vi "Levenberg Marquardt Prep.vi"(0 "Structure":T1 {"?" format="%.2f"; "?" format="%.2f"; "Initial Guess Coefficient" format="%.2f"; "?" format="%.2f"; "X" format="%.2f"; "Parsed Formula copy"."Y Values" format="%.2f"; "Y Values" format="%.2f"; "Y" format="%.2f"; "Parsed Formula"."Y Values" format="%.2f"}, 1 "max iteration":i32=200) -> (2 "Covariance":dbl[][](array[numeric]) format="%.2f", 3 "Best Fit":dbl[](array[numeric]) format="%.2f", 4 "Best Fit Coefficients":dbl[](array[numeric]) format="%.2f", 5 "mse":dbl format="%.2e")   [LabVIEW 2017, in "NI_Gmath.lvlib"]
uses:
  NI_Gmath.lvlib
  Real Outer Product.vi
  Solve Linear Equations (single right hand).vi
  Solve Linear Equations By Cholesky.vi
  Real Matrix to Compact Array.vi
  Real Compact Tri-Matrix Linear Eqs.vi
  Solve Linear Eqs (General).vi
  Solve Linear Eqs (Gen, single right hand).vi
  Add - RM,RM.vi
  Multiply - RM,RM.vi
  Multiply - R,RM.vi
  Create Special Real Matrix.vi
  NI_AALPro.lvlib
  NI_AALBase.lvlib
  NI_Matrix.lvlib
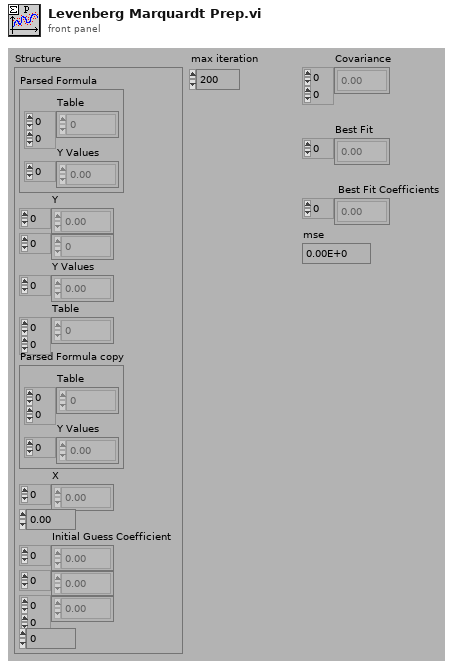
[diagram p1: front panel]
types:
  T1 = cluster{"Parsed Formula":cluster{"Table":i32[][], "Y Values":dbl[]}, "Y":dbl[], i32[], "Y Values":dbl[], "Table":i32[][], "Parsed Formula copy":cluster{"Table":i32[][], "Y Values":dbl[]}, "X":dbl[], dbl, "Initial Guess Coefficient":dbl[], dbl[], dbl[][], i32}
  T2 = enum32{"Identity", "Diagonal", "Toepliz", "Vandermonde", "Companion"}
  T3 = typedef "NI_Matrix.lvlib/RealMatrix.ctl" = dbl[][]
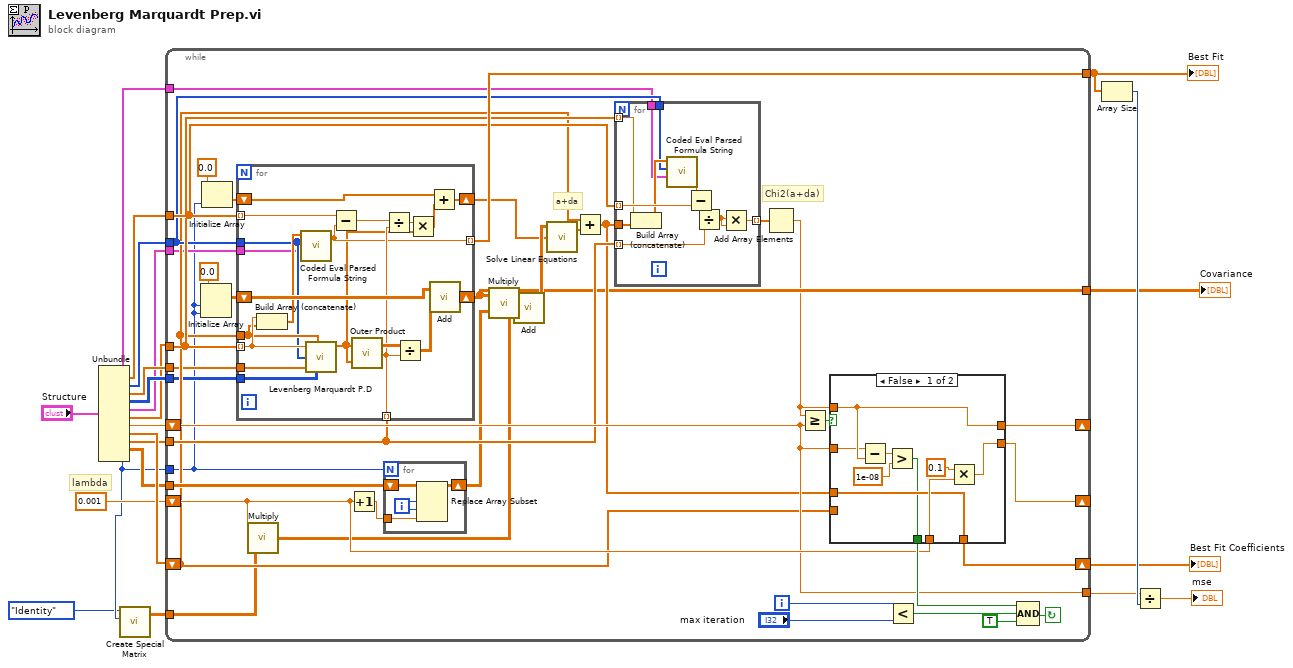
[diagram p0: block diagram]
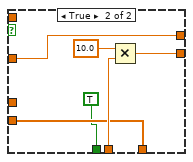
[diagram p2: hidden frame]
diagram:
  # "lambda"
  n1 = Unbundle("Structure") -> ("Parsed Formula"=w11:cluster{"Table":i32[][], "Y Values":dbl[]}, "Y"=w12:dbl[], w13:i32[], "Y Values"=w20:dbl[], "Table"=w19:i32[][], "Parsed Formula copy"=w14:cluster{"Table":i32[][], "Y Values":dbl[]}, "X"=w15:dbl[], w16:dbl, "Initial Guess Coefficient"=w22:dbl[], w17:dbl[], w18:dbl[][], w4:i32)
  n2 = call-poly "Create Special Matrix.vi"("matrix type"=T2."Identity", "matrix size"=w4) -> ("Special Matrix"=w3:T3)  [unwired: 3 in, 1 out]
  n3 = while {
    tunnel: [w29] -> w9
    tunnel: w11 -> [w37]
    tunnel: w14 -> [w38]
    tunnel: [w58] -> w6
    tunnel: [w60] -> w2
    tunnel: w20 -> [w35]
    tunnel: w19 -> [w36]
    tunnel: w13 -> [w43]
    tunnel: w12 -> [w57]
    tunnel: w18 -> [w44]
    tunnel: w4 -> [w31]
    tunnel: w17 -> [w50]
    tunnel: w15 -> [w51]
    shift-left: w16 -> [w60]
    shift-right: [w45] -> _
    shift-left: w22 -> [w40]
    shift-right: [w48] -> w8
    shift-left: 0.001 -> [w61]
    shift-right: [w46] -> _
    tunnel: w3 -> [w26]
    i -> [w32]
    stop <- w33 continue-if-true
    # "Chi2(a+da)"
    # "a+da"
    n4 = Initialize Array(0.0, w31, w31) -> (w55:dbl[][])
    n5 = Initialize Array(0.0, w31) -> (w53:dbl[])
    n6 = for {
      tunnel: w51 -> [w101] mode=indexing
      tunnel: w40 -> [w100]
      tunnel: w50 -> [w106] mode=indexing
      shift-right: [w109] -> w29
      shift-left: w55 -> [w111]
      tunnel: w57 -> [w108] mode=indexing
      shift-right: [w102] -> w39
      shift-left: w53 -> [w107]
      tunnel: w43 -> [w94]
      tunnel: w36 -> [w98]
      tunnel: w35 -> [w99]
      tunnel: [w97] -> w58 mode=indexing
      tunnel: w38 -> [w93]
      n7 = Build Array (concatenate)(w101, w100) -> (w95:dbl[])
      n8 = call "Coded Eval Parsed Formula String.vi"("Parsed Formula"=w93, "Variables"=w94, "X Values"=w95) -> ("y value"=w97:dbl)  [unwired: 1 in, 1 out]
      n9 = call "Levenberg Marquardt P.D.vi"("x"=w101, "A"=w100, "variable"=w94, "result"=w99, "table"=w98) -> ("dy(y,a)/da"=w96:dbl[])
      n10 = Subtract(x=w108, y=w97) -> (x-y=w105:dbl)
      n11 = call-poly "Outer Product.vi"("Y Vector"=w96, "X Vector"=w96) -> ("Outer Product"=w112:T3)  [unwired: 1 out]
      n12 = Divide(x=w105, y=w106) -> (x/y=w104:dbl)
      n13 = Divide(x=w112, y=w106) -> (x/y=w110:T3)
      n14 = Multiply(x=w104, y=w96) -> (x*y=w103:dbl[])
      n15 = Add(x=w107, y=w103) -> (x+y=w102:dbl[])
      n16 = call-poly "Add.vi"("Real Matrix B"=w110, "Real Matrix A"=w111) -> ("A + B"=w109:T3)
    }
    n17 = call-poly "Multiply.vi"("Real Matrix A"=w26, "Real Scalar c"=w61) -> ("c * A"=w25:T3)
    n18 = Increment(x=w61) -> (x+1=w24:dbl)
    n19 = for {
      N: w31 -> [_]
      tunnel: w24 -> [w91]
      shift-right: [w89] -> w41
      shift-left: w44 -> [w90]
      i -> [w92]
      n20 = Replace Array Subset(array=w90, new element=w91, index (row)=w92, index (col)=w92) -> (w89:dbl[][])
    }
    n21 = call-poly "Multiply.vi"("Real Matrix B"=w41, "Real Matrix A"=w29) -> ("A * B"=w23:T3)
    n22 = call-poly "Add.vi"("Real Matrix B"=w25, "Real Matrix A"=w23) -> ("A + B"=w59:T3)
    n23 = call-poly "Solve Linear Equations.vi"("Known Vector"=w39, "Input Matrix"=w59) -> ("Solution Vector"=w52:dbl[])  [unwired: 1 in, 1 out]
    n24 = Add(x=w40, y=w52) -> (x+y=w47:dbl[])
    n25 = for {
      tunnel: w51 -> [w81] mode=indexing
      tunnel: w47 -> [w82]
      tunnel: w57 -> [w88] mode=indexing
      tunnel: w50 -> [w86] mode=indexing
      tunnel: [w84] -> w30 mode=indexing
      tunnel: w43 -> [w79]
      tunnel: w37 -> [w78]
      n26 = Build Array (concatenate)(w81, w82) -> (w80:dbl[])
      n27 = call "Coded Eval Parsed Formula String.vi"("Parsed Formula"=w78, "Variables"=w79, "X Values"=w80) -> ("y value"=w83:dbl)  [unwired: 1 in, 1 out]
      n28 = Subtract(x=w83, y=w88) -> (x-y=w87:dbl)
      n29 = Divide(x=w87, y=w86) -> (x/y=w85:dbl)
      n30 = Multiply(x=w85, y=w85) -> (x*y=w84:dbl)
    }
    n31 = Add Array Elements(numeric array=w30) -> (sum=w27:dbl)
    n32 = Greater Or Equal?(x=w27, y=w60) -> (x >= y?=w49:bool)
    n33 = case shown="False" w49 {
      tunnel: w61 -> [w70 w76]
      tunnel: w40 -> [_ w75]
      tunnel: [w69 w75] -> w48
      tunnel: w47 -> [w69 _]
      tunnel: [w68 w74] -> w46
      tunnel: [w67 w73] -> w45
      tunnel: w60 -> [w66 w73]
      tunnel: w27 -> [w67 _]
      tunnel: [w64 TRUE] -> w62
      frame False {
        n34 = Subtract(x=w66, y=w67) -> (x-y=w63:dbl)
        n35 = Greater?(x=w63, y=1e-08) -> (0:w64:bool)
        n36 = Multiply(x=0.1, y=w70) -> (x*y=w68:dbl)
      }
      frame True {
        n37 = Multiply(x=10.0, y=w76) -> (x*y=w74:dbl)
      }
    }
    n38 = Less?(x=w32, y="max iteration") -> (x < y?=w34:bool)
    n39 = Compound Arithmetic op=AND(w62, w34, TRUE ("value")) -> (w33:bool)
  }
  "Covariance" <- w9
  "Best Fit" <- w6
  "Best Fit Coefficients" <- w8
  n40 = Array Size(array=w6) -> (size(s)=w21:i32)
  n41 = Divide(x=w2, y=w21) -> (x/y=→"mse":dbl)
